vi "SingleSeq.vi"(6 "Motion System":T1=enum."No Motion Card", 8 "GL Ref Out":refnum<k7>, 9 "Motion Bd ID":u8=1 min=1 max=32 step=1, 10 "Digitizer Settings":T2={"Digitizer delay (us) "=0.0, "rf points per line"=2048, "lines per plane"=128, "Samp Rate (Hz)"=100000000.0, "Additional dig delay (us)"=0.0, "Voltage Scale"=0.4, "Pre-Looks"=0, "Offset delay (us)"=0.0, "bits A/D"=8, "Avg Num"=1, "DigTimeOut"=5.0, "Rel Dig Delay"=0.0, "Dig Ch"=0, "LeCroyCluster"={"LeCroy Channels"=[TRUE, FALSE, FALSE, FALSE], "LC read pt offset"=0.0, "Sweep Avg"=FALSE}, "Main Digitizer"=enum."NI Digitizer", "Dig Config"=enum."Single channel", "Digitizer ID Cluster"={"Acqiris/Alazar/SP ID"=[], "NI Instr Handles"=[], "LeCroy VISA"="", "GaGe Handle"={"Handle"=0, "Sample size"=0, "Resolution"=0, "Offset"=0, "Channels"=0, "Boards"=0}, "ATS Ref"="ATS9350", "Acqiris Address"=["PCI::INSTR0"], "ADQRef"=refnum, "adq_cu_ptr"=refnum}, "Trigger Settings"={"Trig Source"=1, "Trig Coupling"=0, "Trig Slope"=0, "Level (mV)"=1500.0}, "Bulk Acq"=FALSE, "Bulk Start Indexes"=[], "Data Ref RF"=refnum, "NI ID/Channel"=[], "Total Dig CH"=5, "Xtra Ann Trig delay (us)"=10.0, "Fix Z Delay?"=FALSE, "One Way Transmission?"=FALSE, "Data Ref Log"=refnum} {"Trigger Settings"."Trig Slope" items=["Positive", "Negative"]; "Trigger Settings"."Level (mV)" format="%.2f"; "Trigger Settings"."Trig Coupling" items=["DC 1 MOhm", "AC 1 MOhm", "DC 50 Ohm", "AC 50 Ohm"]; "Trigger Settings"."Trig Source" items=["Chan 1", "External"]; "Rel Dig Delay" format="%.2f"; "DigTimeOut" format="%.2f"; "Avg Num" min=1; "Offset delay (us)" format="%.2f"; "Additional dig delay (us)" format="%.2f"; "Digitizer delay (us)" format="%.2f"}) -> (0 "Status":i32, 1 "gain":dbl, 2 "errorMessage":string, 3 "waveform":dbl[](array[numeric]) format="%.2e")   [LabVIEW 2022 SP3]
uses:
  -DigitizerRoutines/DigitizerSettings.ctl
  -DigitizerRoutines/Digitizer.ctl
  -DigitizerRoutines/DigConfig.ctl
  -DigitizerRoutines/DigitizerID.ctl
  C:/Windows/System32/ADQAPI_dotNet_helper.dll
  Motion Controllers/NI_controller/-NI_MotionRoutines/MotionSys.ctl
  <vilib>/Analysis/baseanly.llb/Mean (DBL).vi
  <vilib>/DAQmx/create/channels.llb/DAQmx Create Channel (CO-Pulse Generation-Frequency).vi
  <vilib>/DAQmx/configure/timing.llb/DAQmx Timing (Implicit).vi
  <instrlib>/niScope/Acquire/Fetch/niScope Multi Fetch.vi
  <instrlib>/Acqiris Dx/Acqiris Dx.lvlib
  <vilib>/Analysis/NI_AALBase.lvlib
panel:
  out "Acquired Waveform SGL":sgl[][](array[numeric])
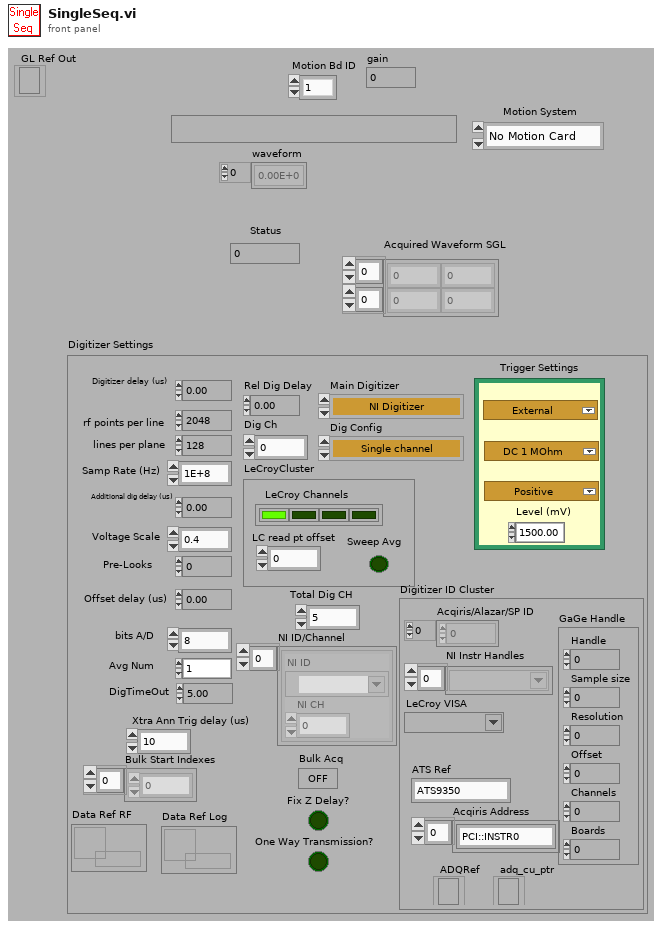
[diagram p1: front panel]
types:
  T1 = typedef "MotionSys.ctl" = enum16{"MM3000", "NI 735x", "Newport ESP", "No Motion Card", "Galil"}
  T2 = typedef "DigitizerSettings.ctl" = cluster{"Digitizer delay (us) ":dbl, "rf points per line":i32, "lines per plane":i32, "Samp Rate (Hz)":dbl, "Additional dig delay (us)":dbl, "Voltage Scale":dbl, "Pre-Looks":i32, "Offset delay (us)":dbl, "bits A/D":i8, "Avg Num":i32, "DigTimeOut":sgl, "Rel Dig Delay":sgl, "Dig Ch":i32, "LeCroyCluster":cluster{"LeCroy Channels":bool[], "LC read pt offset":dbl, "Sweep Avg":bool}, "Main Digitizer":T3, "Dig Config":T4, "Digitizer ID Cluster":T5, "Trigger Settings":cluster{"Trig Source":u16, "Trig Coupling":u16, "Trig Slope":u16, "Level (mV)":dbl}, "Bulk Acq":bool, "Bulk Start Indexes":i32[], "Data Ref RF":refnum<data-value>, "NI ID/Channel":cluster{"NI ID":refnum<k15>, "NI CH":i32}[], "Total Dig CH":i32, "Xtra Ann Trig delay (us)":dbl, "Fix Z Delay?":bool, "One Way Transmission?":bool, "Data Ref Log":refnum<data-value>}
  T3 = typedef "Digitizer.ctl" = enum16{"Acqiris Digitizer", "NI Digitizer", "LeCroy", "GaGe", "AlazarTech", "No Digitizer", "Teledyne"}
  T4 = typedef "DigConfig.ctl" = enum16{"Single channel", "2 Chans w/ 2 Acqiris", "2 Chans w/ 1 Acqiris", "5-CH Pulser New", "5-CH pulser w/ ann array", "5-pass style ann array", "Empty"}
  T5 = typedef "DigitizerID.ctl" = cluster{"Acqiris/Alazar/SP ID":u32[], "NI Instr Handles":refnum<k15>[], "LeCroy VISA":refnum<visa-resource-name>, "GaGe Handle":cluster{"Handle":u32, "Sample size":u32, "Resolution":i32, "Offset":i32, "Channels":u32, "Boards":u32}, "ATS Ref":string, "Acqiris Address":string[], "ADQRef":refnum<k24>, "adq_cu_ptr":refnum<k24>}
  T6 = cluster{"actualSamples":i32, "absoluteInitialX":dbl, "relativeInitialX":dbl, "xIncrement":dbl, "offset":dbl, "gain":dbl, "reserved1":dbl, "reserved2":dbl}[]
  T7 = cluster{"actualSamples":i32, "absoluteInitialX":dbl, "relativeInitialX":dbl, "xIncrement":dbl, "offset":dbl, "gain":dbl, "reserved1":dbl, "reserved2":dbl}
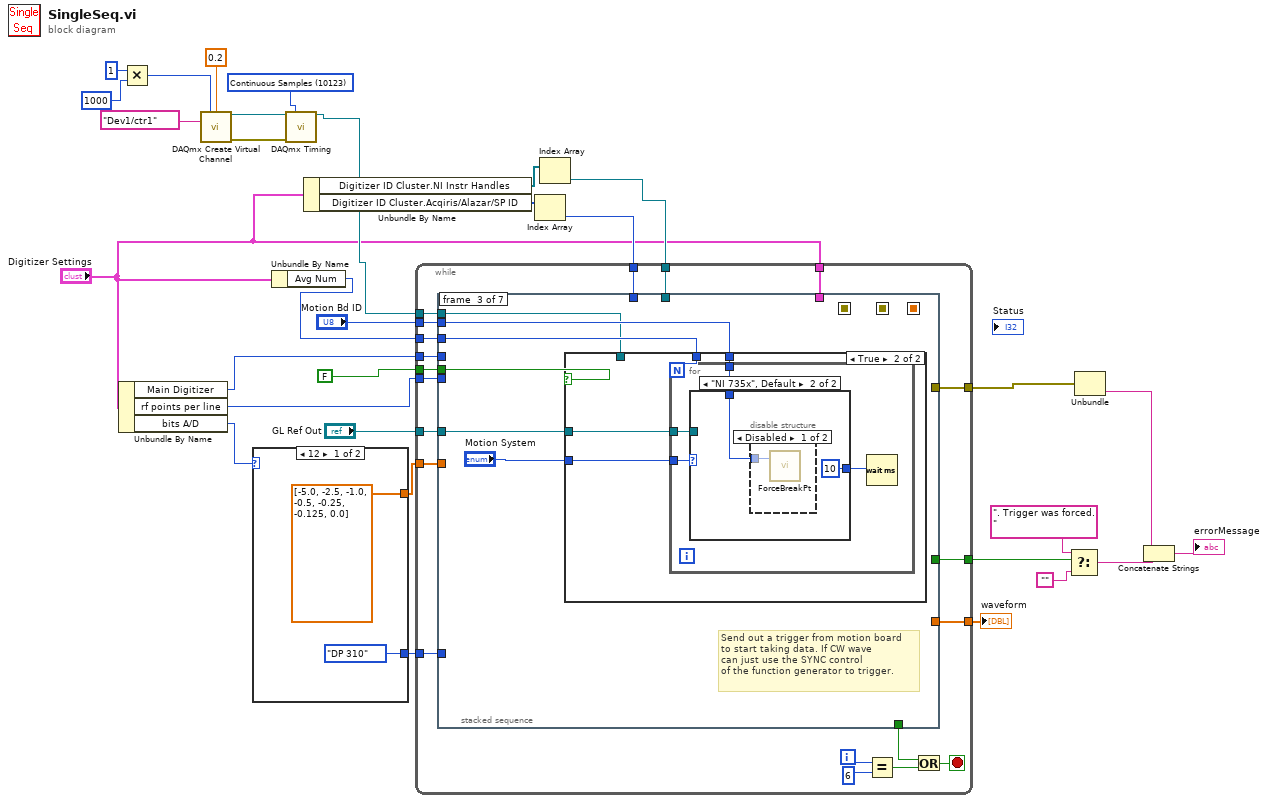
[diagram p0: block diagram]
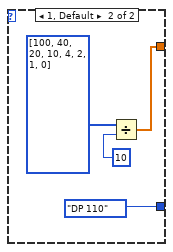
[diagram p2: hidden frame]
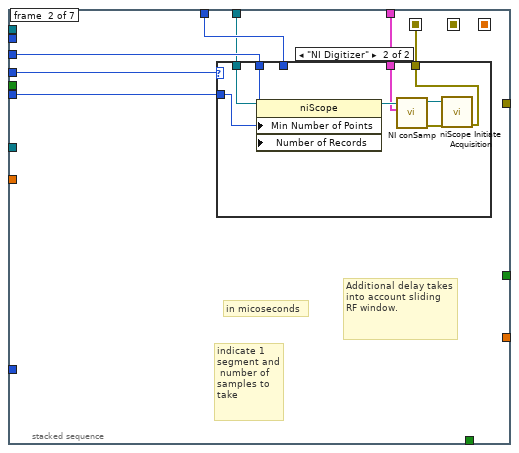
[diagram p4: hidden frame]
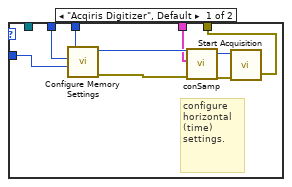
[diagram p5: hidden frame]
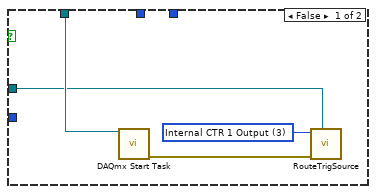
[diagram p6: hidden frame]
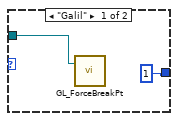
[diagram p7: hidden frame]
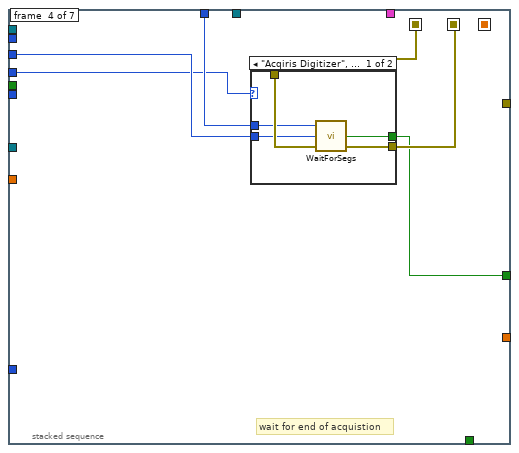
[diagram p9: hidden frame]
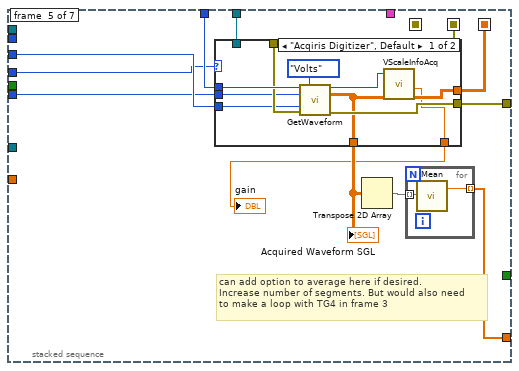
[diagram p11: hidden frame]
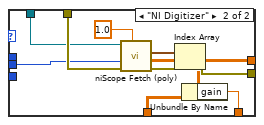
[diagram p12: hidden frame]
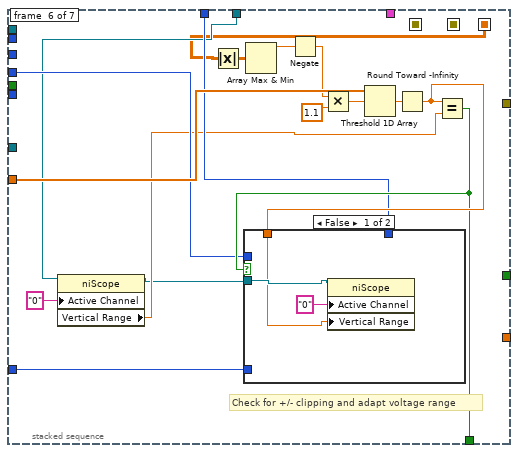
[diagram p13: hidden frame]
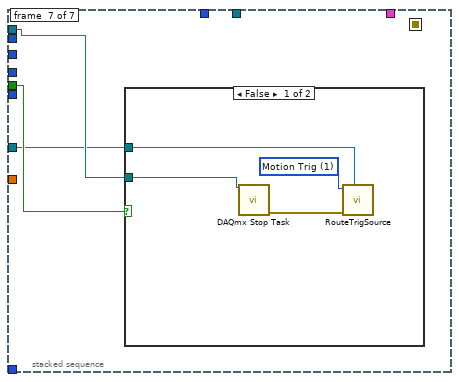
[diagram p15: hidden frame]
diagram:
  w8 = 10123 items=["Finite Samples"=10178, "Continuous Samples"=10123] ("sample mode")
  n1 = Unbundle By Name("Digitizer Settings") -> ("Main Digitizer"=w3:T3, "rf points per line"=w6:i32, "bits A/D"=w2:i8)
  n2 = Multiply(x=1, y=1000) -> (x*y=w12:i32)
  n3 = call-poly <vilib>:"DAQmx Create Virtual Channel.vi"("frequency"=w12, "duty cycle"=0.2, "counter"=tag "Dev1/ctr1") -> ("task out"=w14:refnum<k21>, "error out"=w15:errorcluster)  [unwired: 11 in]
  n4 = case shown="12" w2 {
    tunnel: [sgl[] [-5.0, -2.5, -1.0, -0.5, -0.25, -0.125, 0.0] w34] -> w26
    tunnel: [enum16{"DP 110", "DP 310"}."DP 310" ("Card Type") enum16{"DP 110", "DP 310"}."DP 110" ("Card Type")] -> w25
    frame 12 {
    }
    frame 1, Default {
      n5 = Divide(x=i32[] [100, 40, 20, 10, 4, 2, 1, 0] ("32bit integer"), y=10) -> (x/y=w34:dbl[])
    }
  }
  n6 = Unbundle By Name("Digitizer Settings") -> ("Avg Num"=w4:i32)
  n7 = call-poly <vilib>:"DAQmx Timing.vi"("task/channels in"=w14, "sample mode"=w8, "error in"=w15) -> ("task out"=w7:refnum<k21>)  [unwired: 11 in, 1 out]
  n8 = Unbundle By Name("Digitizer Settings") -> ("Digitizer ID Cluster.NI Instr Handles"=w20:refnum<k15>[], "Digitizer ID Cluster.Acqiris/Alazar/SP ID"=w19:u32[])
  n9 = Index Array(array=w19) -> (element=w18:u32)  [unwired: 1 in]
  n10 = Index Array(array=w20) -> (element=w17:refnum<k15>)  [unwired: 1 in]
  n11 = while {
    tunnel: [w57] -> w27
    tunnel: w4 -> [w56]
    tunnel: [w55] -> w22
    tunnel: w6 -> [w54]
    tunnel: w18 -> [w53]
    tunnel: [w52] -> w23
    tunnel: w26 -> [w51]
    tunnel: w25 -> [w45]
    tunnel: "Motion Bd ID" -> [w44]
    tunnel: w3 -> [w43]
    tunnel: w17 -> [w42]
    tunnel: FALSE -> [w41]
    tunnel: w7 -> [w40]
    tunnel: "Digitizer Settings" -> [w39]
    tunnel: "GL Ref Out" -> [w38]
    i -> [w49]
    stop <- w46 stop-if-true
    n12 = stacked-sequence {
      seq-local: [_ _ _ w109 _ _ _] -> [_ _ _ _ w127 _ _]
      seq-local: [_ w64 _ _ _ _ _] -> [_ _ _ w110 _ _ _]
      seq-local: [_ _ _ _ w118 _ _] -> [_ _ _ _ _ w150 _]
      tunnel: w53 -> [_ w63 _ w108 w128 w158 _]
      tunnel: [_ _ _ w106 _ _ _] -> w57
      tunnel: w56 -> [_ w62 w87 w107 w125 _ _]
      tunnel: w54 -> [_ w61 _ _ w124 _ _]
      tunnel: [_ _ _ _ w126 _ _] -> w55
      tunnel: [_ _ _ _ w121 _ _] -> w52
      tunnel: w51 -> [_ _ _ _ _ w162 _]
      tunnel: [_ _ _ _ _ w160 _] -> w47
      tunnel: w45 -> [_ _ _ _ _ w159 _]
      tunnel: w44 -> [_ _ w86 _ _ _ _]
      tunnel: w43 -> [_ w60 _ w105 w120 w157 _]
      tunnel: w42 -> [_ w59 _ _ w119 w154 _]
      tunnel: w41 -> [_ _ w85 _ _ _ w171]
      tunnel: w40 -> [_ _ w84 _ _ _ w170]
      tunnel: w39 -> [_ w58 _ _ _ _ _]
      tunnel: w38 -> [_ _ w82 _ _ _ w169]
      frame #0 {
      }
      frame #1 {
        # "indicate 1 segment and\n number of samples to take"
        # "Additional delay takes into account sliding\nRF window."
        # "in micoseconds"
        n13 = case shown="\"NI Digitizer\"" w60 {
          tunnel: [w71 w75] -> w64
          tunnel: w63 -> [w69 _]
          tunnel: w62 -> [w67 w80]
          tunnel: w61 -> [w66 w81]
          tunnel: w59 -> [_ w79]
          tunnel: w58 -> [w65 w74]
          frame "Acqiris Digitizer", Default {
            # "configure horizontal (time)\nsettings."
            n14 = call <instrlib>:"Configure Memory Settings.vi"("Number of Samples (1000)"=w66, "Number of Segments (1)"=w67, "Instrument ID"=w69) -> ("error out"=w68:errorcluster, "dup Instrument ID"=w70:u32)  [unwired: 1 in, 2 out]
            n15 = call "conSamp.vi"("error in"=w68, "Digitizer Settings"=w65, "InstrumentID"=w70) -> ("error out"=w72:errorcluster, "DUP ID"=w73:u32)  [unwired: 1 in]
            n16 = call <instrlib>:"Start Acquisition.vi"("error in (no error)"=w72, "Instrument ID"=w73) -> ("error out"=w71:errorcluster)  [unwired: 2 in, 1 out]
          }
          frame "NI Digitizer" {
            n17 = property class="niScope"(reference=w79, "Min Number of Points"=w81, "Number of Records"=w80) -> (reference out=w78:refnum<k15>)  [unwired: 1 in, 1 out]
            n18 = call "NI conSamp.vi"("Digitizer Settings"=w74, "InstrumentID"=w78) -> ("error out"=w76:errorcluster, "DUP ID"=w77:refnum<k15>)  [unwired: 2 in]
            n19 = call <instrlib>:"niScope Initiate Acquisition.vi"("instrument handle"=w77, "error in"=w76) -> ("error out"=w75:errorcluster)  [unwired: 13 out]
          }
        }
      }
      frame #2 {
        # "Send out a trigger from motion board\nto start taking data. If CW wave\ncan just use the SYNC control\nof the function generator to trigger."
        n20 = case shown="True" w85 {
          tunnel: "Motion System" -> [_ w95]
          tunnel: w87 -> [_ w94]
          tunnel: w86 -> [_ w93]
          tunnel: w84 -> [w89 _]
          tunnel: w82 -> [w88 w92]
          frame False {
            w90 = u16 3 items=["Function Gen Input", "Motion Trig", "Internal RT Motion Trig", "Internal CTR 1 Output"] ("Trig Source")
            n21 = call <vilib>:"DAQmx Start Task.vi"("task/channels in"=w89) -> ("error out"=w91:errorcluster)  [unwired: 13 in, 1 out]
            n22 = call "RouteTrigSource.vi"("Galil.IGalil"=w88, "error in"=w91, "Trig Source"=w90) -> ()  [unwired: 8 in, 1 out]
          }
          frame True {
            n23 = for {
              N: w94 -> [_]
              tunnel: w95 -> [w97]
              tunnel: w93 -> [w98]
              tunnel: w92 -> [w96]
              n24 = case shown="\"NI 735x\", Default" w97 {
                tunnel: [1 10] -> w99
                tunnel: w98 -> [_ w102]
                tunnel: w96 -> [w100 _]
                frame "Galil" {
                  n25 = call "GL_ForceBreakPt.vi"("GL Ref Out"=w100) -> ()  [unwired: 1 in, 2 out]
                }
                frame "NI 735x", Default {
                  n26 = disable-structure shown="Disabled" {
                    disable-tunnel: w102 -> [w104 _]
                    frame Disabled {
                      n27 = call "ForceBreakPt.vi"("Bd ID in"=w104) -> ()  [unwired: 1 in, 2 out]
                    }
                    frame Enabled {
                    }
                  }
                }
              }
              n28 = Wait (ms)(milliseconds to wait=w99) -> ()  [unwired: 1 out]
            }
          }
        }
      }
      frame #3 {
        # "wait for end of acquistion"
        n29 = case shown="\"Acqiris Digitizer\", Default" w105 {
          tunnel: w110 -> [w115 w116]
          tunnel: [w114 w116] -> w109
          tunnel: w108 -> [w113 _]
          tunnel: w107 -> [w112 _]
          tunnel: [w111 _] -> w106
          frame "Acqiris Digitizer", Default {
            n30 = call "WaitForSegs.vi"("Acqiris ID"=w113, "lines per plane"=w112, "error in"=w115) -> ("status"=w111:bool, "error out"=w114:errorcluster)  [unwired: 1 in, 2 out]
          }
          frame "NI Digitizer" {
          }
        }
      }
      frame #4 {
        # "can add option to average here if desired.\nIncrease number of segments. But would also need\nto make a loop with TG4 in frame 3"
        n31 = case shown="\"Acqiris Digitizer\", Default" w120 {
          tunnel: w128 -> [w137 _]
          tunnel: w127 -> [w136 w146]
          tunnel: [w135 w143] -> w126
          tunnel: w125 -> [w134 _]
          tunnel: w124 -> [w133 w144]
          tunnel: [w131 w142] -> w122
          tunnel: w119 -> [_ w145]
          tunnel: [w131 w142] -> w118
          tunnel: [w129 w138] -> w117
          frame "Acqiris Digitizer", Default {
            n32 = call "GetWaveform.vi"("Acq ID Out"=w137, "Read Mode"=enum32{"ADC", "Volts"}."Volts", "Num Samps"=w133, "Num Segs"=w134, "error in"=w136) -> ("Acq ID Out"=w130:u32, "Acquired Waveform SGL"=w131:dbl[][], "error out"=w135:errorcluster)  [unwired: 1 in, 7 out]
            n33 = call "VScaleInfoAcq.vi"("Instrument ID"=w130) -> ("Total Gain (dB)"=w129:dbl)  [unwired: 6 in, 3 out]
          }
          frame "NI Digitizer" {
            n34 = call-poly <instrlib>:"niScope Fetch (poly).vi"("timeout"=1.0, "error in"=w146, "numSamples"=w144, "instrument handle"=w145) -> ("error out"=w143:errorcluster, "wfm"=w142:dbl[][], "wfm info"=w140:T6)  [unwired: 1 in, 4 out]
            n35 = Index Array(array=w140) -> (element=w139:T7)  [unwired: 1 in]
            n36 = Unbundle By Name(w139) -> ("gain"=w138:dbl)
          }
        }
        "Acquired Waveform SGL" <- w122
        "gain" <- w117
        n37 = Transpose 2D Array(2D array=w122) -> (transposed array=w123:dbl[][])
        n38 = for {
          tunnel: w123 -> [w147] mode=indexing
          tunnel: [w148] -> w121 mode=indexing
          n39 = call-poly <vilib>:"Mean.vi"("X"=w147) -> ("mean"=w148:dbl)  [unwired: 1 out]
        }
      }
      frame #5 {
        # "Check for +/- clipping and adapt voltage range"
        n40 = property class="niScope"(reference=w154, "Active Channel"="0") -> (reference out=w153:refnum<k15>, "Vertical Range"=w155:dbl)  [unwired: 1 in, 1 out]
        n41 = Absolute Value(x=w150) -> (abs(x)=w152:dbl[][])
        n42 = Array Max & Min(array=w152) -> (max value=w151:dbl)  [unwired: 3 out]
        n43 = Negate(x=w151) -> (-x=w149:dbl)
        n44 = Multiply(x=w149, y=1.1) -> (x*y=w165:dbl)
        n45 = Threshold 1D Array(2:w165, 3:w162) -> (0:w163:dbl)  [unwired: 1 out]
        n46 = Round Toward -Infinity(1:w163) -> (0:w161:dbl)
        n47 = Equal?(x=w161, y=w155) -> (x = y?=w160:bool)
        n48 = case shown="False" w160 {
          tunnel: w161 -> [w167 _]
          tunnel: w159 -> [_ _]
          tunnel: w158 -> [_ _]
          tunnel: w157 -> [_ _]
          tunnel: w153 -> [w168 _]
          frame False {
            n49 = property class="niScope"(reference=w168, "Active Channel"="0", "Vertical Range"=w167) -> ()  [unwired: 1 in, 2 out]
          }
          frame True {
          }
        }
      }
      frame #6 {
        n50 = case shown="False" w171 {
          tunnel: w170 -> [w173 _]
          tunnel: w169 -> [w172 _]
          frame False {
            w175 = u16 1 items=["Function Gen Input", "Motion Trig", "Internal RT Motion Trig", "Internal CTR 1 Output"] ("Trig Source")
            n51 = call <vilib>:"DAQmx Stop Task.vi"("task/channels in"=w173) -> ("error out"=w174:errorcluster)  [unwired: 13 in, 1 out]
            n52 = call "RouteTrigSource.vi"("Galil.IGalil"=w172, "error in"=w174, "Trig Source"=w175) -> ()  [unwired: 8 in, 1 out]
          }
          frame True {
          }
        }
      }
    }
    n53 = Equal?(x=w49, y=6) -> (x = y?=w48:bool)
    n54 = Or(x=w47, y=w48) -> (x .or. y?=w46:bool)
  }
  "waveform" <- w23
  n55 = Select(t=". Trigger was forced.", s=w27, f="") -> (s? t:f=w29:string)
  n56 = Unbundle(w22) -> ("source"=w21:string)  [unwired: 2 out]
  n57 = Concatenate Strings(w21, w29) -> (→"errorMessage":string)
